vi "uActor_Send to Self (High Priority).vi"(8 "error in (no error)":errorcluster, 10 "uMsg":refnum<class "uMsg.lvclass">, 11 "uActor in":refnum<class "uActor.lvclass">) -> (0 "error out":errorcluster, 3 "uActor out":refnum<class "uActor.lvclass">)   [LabVIEW 2021, in "uFramework.lvlib" / "uActor.lvclass"]
doc: "Use by an actor to enqueue a message to self at the FRONT of the message queue."
uses:
  uActor.lvclass
  uMsg/uMsg.lvclass
  uActor.lvclass/uActor.ctl
  uMsg/uMsg.lvclass/uMsg.ctl
  uTransport_uActor/uTransport_uActor.lvclass/uTransport_uActor.ctl
  uTransport_uActor/uTransport_uActor_SendMsg.vi
  uMsg/uMsg Update Timestamp.vi
  uTransport_uActor/uTransport_uActor.lvclass
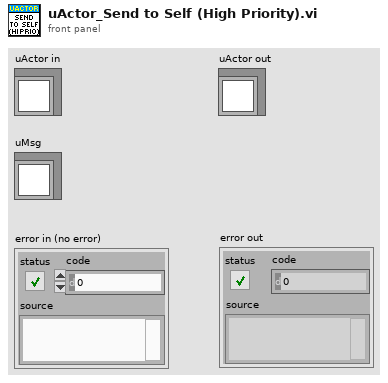
[diagram p1: front panel]
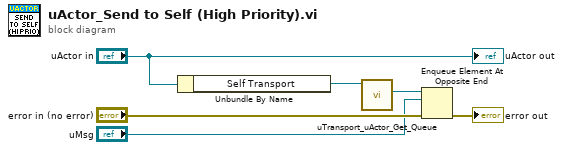
[diagram p0: block diagram]
diagram:
  n1 = Unbundle By Name("uActor in") -> ("Self Transport"=w4:refnum<class "uTransport_uActor.lvclass">)
  n2 = call "uTransport_uActor_Get_Queue.vi"("uTransport_uActor in"=w4) -> ("Actor Queue"=w3:refnum<queue>)  [unwired: 10 in]
  n3 = Enqueue Element At Opposite End(queue=w3, element="uMsg", error in (no error)="error in (no error)") -> (error out=→"error out":errorcluster)  [unwired: 1 in, 2 out]
  "uActor out" <- "uActor in"
